vi "Init Hardware.vi"(8 "error in (no error)":errorcluster, 11 "LR-700 Driver in":refnum<class "LR-700 Driver.lvclass">) -> (0 "error out":errorcluster, 3 "LR-700 Driver out":refnum<class "LR-700 Driver.lvclass">)   [LabVIEW 2019, in "LR-700 Driver.lvclass"]
uses:
  LR-700 Driver.lvclass
  C:/GitHub/NHMFL_Core/Libraries/Instruments/Instrument Driver/Instrument Driver.lvclass
  Instrument Driver/Instrument Driver.lvclass/Instrument Driver.ctl
  Instrument Driver/Read Recorder name.vi
  Instrument Driver/Write Channel names.vi
  Instrument Driver/Write Channel units.vi
  Instrument Driver/Channel Scanner Driver/Channel Scanner Driver.lvclass
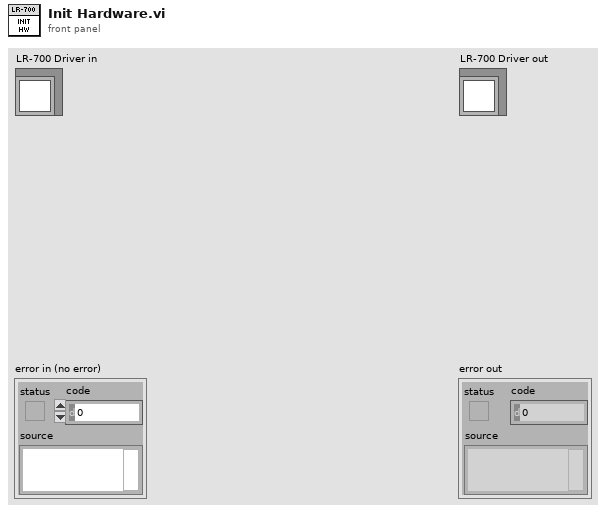
[diagram p1: front panel]
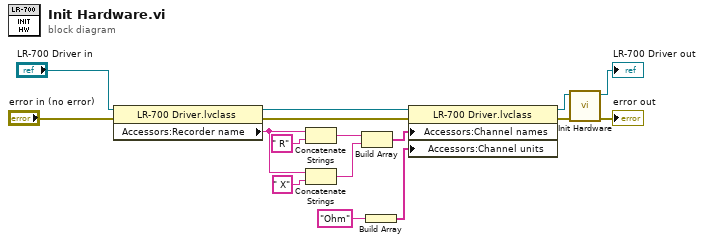
[diagram p0: block diagram]
diagram:
  n1 = property class="LR-700 Driver.lvclass"(reference="LR-700 Driver in", error in="error in (no error)") -> (reference out=w12:refnum<class "LR-700 Driver.lvclass">, error out=w13:errorcluster, "Accessors:Recorder name"=w6:string)
  n2 = Concatenate Strings(w6, " R") -> (w14:string)
  n3 = Concatenate Strings(w6, " X" ("string")) -> (w7:string)
  n4 = Build Array(w14, w7) -> (w9:string[])
  n5 = Build Array("Ohm") -> (w11:string[])
  n6 = property class="LR-700 Driver.lvclass"(reference=w12, error in=w13, "Accessors:Channel names"=w9, "Accessors:Channel units"=w11) -> (reference out=w2:refnum<class "LR-700 Driver.lvclass">, error out=w1:errorcluster)
  n7 = call-parent "Init Hardware.vi"("error in (no error)"=w1, "Instrument Driver in"=w2) -> ("error out"=→"error out":errorcluster, "Instrument Driver out"=→"LR-700 Driver out":refnum<class "LR-700 Driver.lvclass">)  [unwired: 8 in]
